vi "실습 9-1.vi"   [LabVIEW 2014]
types:
  T1 = enum16{"open", "replace", "create", "open or create", "replace or create", "replace or create with confirmation"}
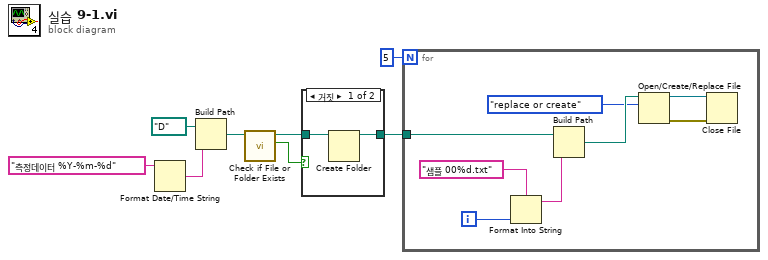
[diagram p0: block diagram]
diagram:
  n1 = Format Date/Time String(time format string (%c)="측정데이터 %Y-%m-%d" ("시간 포맷 문자열 (%c)")) -> (date/time string=w1:string)  [unwired: 2 in]
  n2 = Build Path(base path=path "D:/" ("베이스 경로"), name or relative path=w1) -> (appended path=w8:path)
  n3 = call <vilib>:"Check if File or Folder Exists.vi"("path"=w8) -> ("file or folder exists?"=w6:bool, "dup path"=w7:path)  [unwired: 8 in, 1 out]
  n4 = case shown="거짓" w6 {
    tunnel: w7 -> [w10 w11]
    tunnel: [w9 w11] -> w4
    frame False {
      n5 = Create Folder(path (use dialog)=w10) -> (created path=w9:path)  [unwired: 2 in, 2 out]
    }
    frame True {
    }
  }
  n6 = for {
    N: 5 -> [_]
    tunnel: w4 -> [w19]
    i -> [w17]
    n7 = Format Into String(format string="샘플 00%d.txt" ("포맷 문자열"), w17) -> (resulting string=w16:string)  [unwired: 2 in, 1 out]
    n8 = Build Path(base path=w19, name or relative path=w16) -> (appended path=w13:path)
    n9 = Open/Create/Replace File(file path (use dialog)=w13, operation (0:open)=T1."replace or create" ("동작(0:open)")) -> (refnum out=w15:refnum<file>, error out=w14:errorcluster)  [unwired: 4 in, 1 out]
    n10 = Close File(refnum=w15, error in=w14) -> ()  [unwired: 2 out]
  }
